vi "XNET Database Open (Subframe).vi"(0 "subframe in":refnum<k21>, 11 "error in (no error)":errorcluster) -> (4 "subframe out":refnum<k21>, 15 "error out":errorcluster)   [LabVIEW 2018]
doc: "Opens a subframe from a database file."
uses:
  nixlvapi.dll
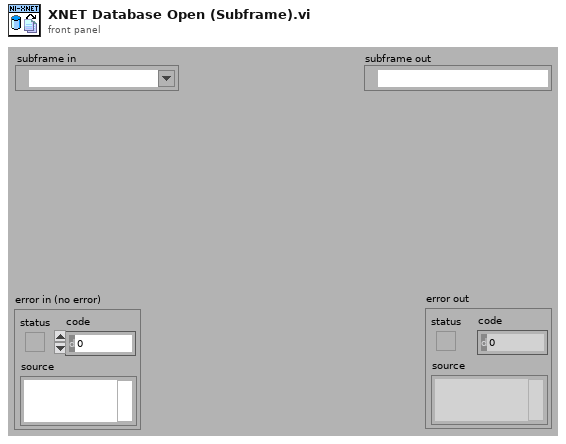
[diagram p1: front panel]
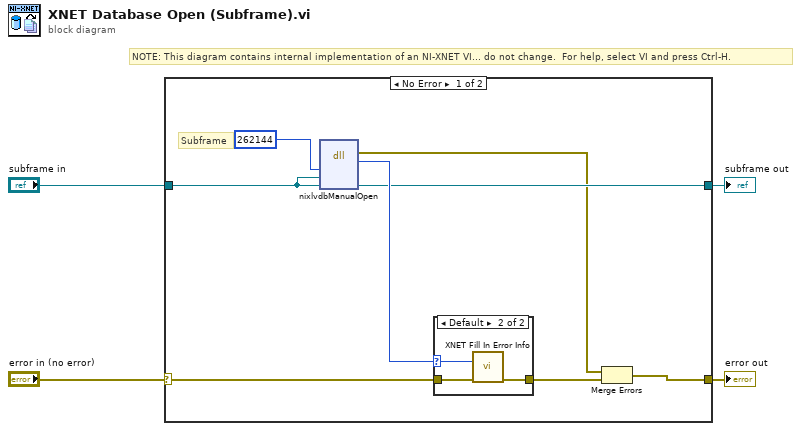
[diagram p0: block diagram]
diagram:
  # "NOTE: This diagram contains internal implementation of an NI-XNET VI... do not change.  For help, select VI and press Ctrl-H."
  n1 = case shown="No Error" "error in (no error)" {
    selector: "error in (no error)" -> [w11 w18]
    tunnel: "subframe in" -> [w8 w17]
    tunnel: [w6 w18] -> w4
    tunnel: [w7 w17] -> w2
    frame No Error {
      # "Subframe"
      n2 = dll-call lib="nixlvapi.*" fn="nixlvdbManualOpen"("objectClass"=u32 262144 ("class"), "lvObjectName"=w8, "output param"=w8) -> (error out=w5:errorcluster, "return type"=w10:i32, "output param"=w7:refnum<k21>)  [unwired: 4 in, 2 out]
      n3 = case shown="Default" w10 {
        selector: w10 -> [_ w14]
        tunnel: w11 -> [w13 w15]
        tunnel: [w13 w16] -> w12
        frame 0 {
        }
        frame Default {
          n4 = call "XNET Fill In Error Info.vi"("status code"=w14, "error in"=w15) -> ("error out"=w16:errorcluster)  [unwired: 13 out]
        }
      }
      n5 = Merge Errors(w5, w12) -> (w6:errorcluster)
    }
    frame Error {
    }
  }
  "error out" <- w4
  "subframe out" <- w2
